vi "tcpExampleClient.vi"() -> ()   [LabVIEW 2014]
uses:
  typedefs/clientStatus.ctl
  typedefs/clientConfiguration.ctl
panel:
  out "client status":T1
  out "receive server->client":string
  in  "transmit client->server":string
  in  "stop":bool
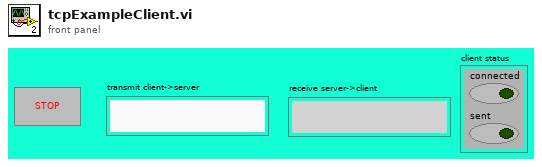
[diagram p1: front panel]
types:
  T1 = typedef "clientStatus.ctl" = cluster{"connected":bool, "sent":bool}
  T2 = typedef "clientConfiguration.ctl" = cluster{"client ID":string, "remote host":string, "local port":u16, "remote port":u16}
  T3 = cluster{"status":cluster{"queue":refnum<queue>, "error out":errorcluster}, "receive":cluster{"queue":refnum<queue>, "error out":errorcluster}, "transmit":cluster{"queue":refnum<queue>, "error out":errorcluster}, "shutdown":cluster{"queue":refnum<queue>, "error out":errorcluster}}
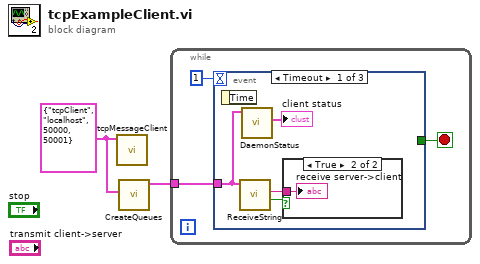
[diagram p0: block diagram]
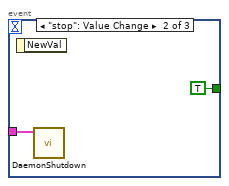
[diagram p3: hidden frame]
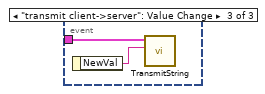
[diagram p4: hidden frame]
diagram:
  w2 = T2 {"client ID"="tcpClient", "remote host"="localhost", "local port"=50000, "remote port"=50001} ("client configuration")
  n1 = call "tcpMessageClient.vi"("client configuration"=w2) -> ()  [unwired: 10 in, 1 out]
  n2 = call "CreateQueues.vi"("client configuration"=w2) -> ("output cluster"=w1:T3)  [unwired: 10 in]
  n3 = while {
    tunnel: w1 -> [w4]
    stop <- w5 stop-if-true
    n4 = event shown="[0] Timeout" {
      selector: _ -> [_ _ _]
      dyn-events: _ -> [_ _ _]
      timeout: 1 -> [_ _ _]
      tunnel: [_ TRUE _] -> w5
      tunnel: w4 -> [w6 w11 w13]
      event Timeout {
        n5 = event-data() -> ()  [unwired: 1 in, 1 out]
        n6 = call "ReceiveString.vi"("queue cluster"=w6) -> ("new value"=w7:bool, "received string"=w9:string)  [unwired: 7 in, 2 out]
        n7 = call "DaemonStatus.vi"("queue cluster"=w6) -> ("status"=→"client status":T1)  [unwired: 8 in, 2 out]
        n8 = case shown="True" w7 {
          tunnel: w9 -> [_ w10]
          frame False {
          }
          frame True {
            "receive server->client" <- w10
          }
        }
      }
      event "stop": Value Change {
        n9 = event-data() -> ()  [unwired: 1 in, 1 out]
        n10 = call "DaemonShutdown.vi"("queue cluster"=w11) -> ()  [unwired: 9 in, 2 out]
      }
      event "transmit client->server": Value Change {
        n11 = event-data() -> ("NewVal"=w14:string)  [unwired: 1 in]
        n12 = call "TransmitString.vi"("string to transmit"=w14, "queue cluster"=w13) -> ()  [unwired: 8 in, 2 out]
      }
    }
  }
